vi "Do.vi"(8 "error in (no error)":errorcluster, 10 "Actor in":refnum<class "Actor.lvclass">, 11 "ReplayData Message":refnum<class "ReplayData Msg.lvclass">) -> (0 "error out":errorcluster, 2 "Actor out":refnum<class "Actor.lvclass">)   [LabVIEW 2014, in "ReplayData Msg.lvclass"]
doc: "(<B>Filename</B>: Actor Framework.lvlib:Message.lvclass:Do.vi)\n\nDefines what a message does when it is received by an actor. Generally, a message instructs an actor to invoke one of its methods. By default, this method does nothing. A child class must override it to define behavior. Create a child class by using the Actor Framework Message Maker dialog box."
uses:
  ReplayData Msg.lvclass
  Data Msg/Data Msg.lvclass
  <vilib>/ActorFramework/Message Enqueuer/Message Enqueuer.lvclass
  ExperimentService/Replay Msg.lvclass
  <vilib>/ActorFramework/Actor/Actor.lvclass
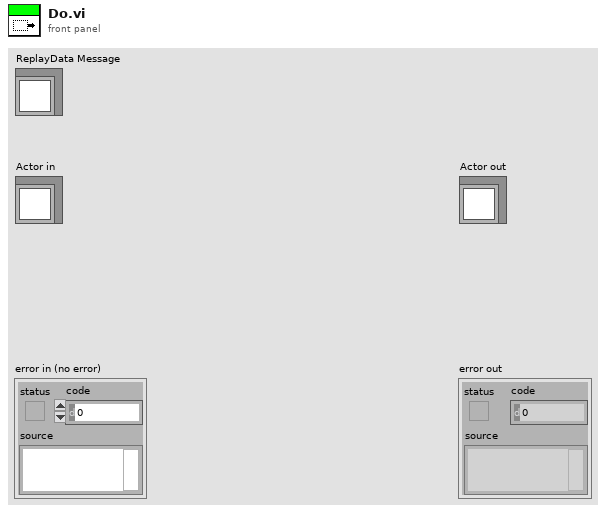
[diagram p1: front panel]
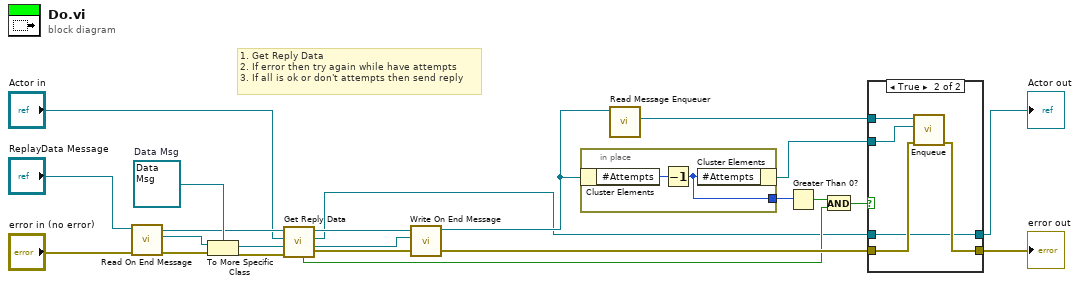
[diagram p0: block diagram]
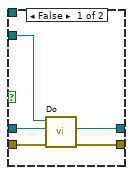
[diagram p2: hidden frame]
diagram:
  w18 = refnum<class "Data Msg.lvclass"> refnum  # Data Msg
  # "1. Get Reply Data\n2. If error then try again while have attempts\n3. If all is ok or don't attempts then send reply"
  n1 = call-dynamic "Read On End Message.vi"("error in (no error)"="error in (no error)", "Replay Msg in"="ReplayData Message") -> ("error out"=w19:errorcluster, "On End Message"=w20:refnum<class "Message.lvclass">, "Replay Msg out"=w14:refnum<class "ReplayData Msg.lvclass">)  [unwired: 7 in]
  n2 = To More Specific Class(target class=w18, reference=w20, error in=w19) -> (specific class reference=w17:refnum<class "Data Msg.lvclass">, error out=w16:errorcluster)
  n3 = call-dynamic "Get Reply Data.vi"("error in (no error)"=w16, "Data Msg in"=w17, "Actor in"="Actor in", "Replay Message"=w14) -> ("error out"=w15:errorcluster, "Data Msg out"=w6:refnum<class "Data Msg.lvclass">, "Actor out"=w1:refnum<class "Actor.lvclass">, "Replay Message out"=w7:refnum<class "ReplayData Msg.lvclass">, "error?"=w8:bool)  [unwired: 3 in]
  n4 = call-dynamic "Write On End Message.vi"("Actor Framework:Message"=w6, "Replay Msg in"=w7) -> ("Replay Msg out"=w4:refnum<class "ReplayData Msg.lvclass">)  [unwired: 8 in, 1 out]
  n5 = in-place {
    in-place-border: [w23] -> w11
    n6 = in-place-cluster #1(w4) -> ("#Attempts"=w24:u32)
    n7 = Decrement(x=w24) -> (x-1=w23:u32)
    n8 = in-place-cluster #1("#Attempts"=w23) -> (w12:refnum<class "ReplayData Msg.lvclass">)
  }
  n9 = call-dynamic "Read Message Enqueuer.vi"("Replay Msg in"=w4) -> ("Actor Framework:Message Enqueuer"=w5:refnum<class "Message Enqueuer.lvclass">)  [unwired: 8 in, 2 out]
  n10 = Greater Than 0?(x=w11) -> (x > 0?=w9:bool)
  n11 = And(x=w9, y=w8) -> (x .and. y?=w10:bool)
  n12 = case shown="True" w10 {
    tunnel: w5 -> [_ w34]
    tunnel: w12 -> [w29 w33]
    tunnel: w15 -> [w27 w32]
    tunnel: [w26 w31] -> w22
    tunnel: [w28 w30] -> w3
    tunnel: w1 -> [w25 w30]
    frame False {
      n13 = call-parent "Do.vi"("error in (no error)"=w27, "Actor in"=w25, "Replay Message"=w29) -> ("error out"=w26:errorcluster, "Actor out"=w28:refnum<class "Actor.lvclass">)  [unwired: 7 in]
    }
    frame True {
      n14 = call <vilib>:"Enqueue.vi"("error in (no error)"=w32, "Message"=w33, "Message Enqueuer in"=w34) -> ("error out"=w31:errorcluster)  [unwired: 7 in, 1 out]
    }
  }
  "error out" <- w22
  "Actor out" <- w3
